vi "WinHostTocRIO.vi"() -> ()   [LabVIEW 2013]
uses:
  <vilib>/userdefined/High Color/nirio_resource_hc.ctl
  <vilib>/nisyscfg/Find Hardware.vi
  <vilib>/nisyscfg/Close (System).vi
  <vilib>/FPGAPlugInAG/NI 9159/niLvFpga_Open_NI 9159.vi
  <vilib>/rvi/interface/common/dynamic/niFpgaDynamicAddResources.vi
  <vilib>/FPGAPlugInAG/Dynamic/niLvFpga_Reset_Dynamic.vi
  <vilib>/FPGAPlugInAG/Dynamic/niLvFpga_Run_Dynamic.vi
  <vilib>/rvi/interface/common/niFpgaWaitOnOcc.vi
  <vilib>/Utility/error.llb/Error Cluster From Error Code.vi
  <vilib>/rvi/errors/niLvFpgaAdjustHostInterfaceError.vi
  <vilib>/FPGAPlugInAG/Dynamic/niLvFpga_Close_Dynamic.vi
  <vilib>/rvi/interface/nirviOpenFPGA/nirviOpenFPGA.xnode
  FPGA Bitfiles/cRIO9159_cRIOIO_v1_1.lvbitx
  cRIO9159_IO.vi
  <vilib>/rvi/interface/nirviMethod/nirviMethod.xnode
  <vilib>/rvi/interface/nirviReadWriteControl/nirviReadWriteControl.xnode
  <vilib>/rvi/interface/nirviCloseFPGA/nirviCloseFPGA.xnode
  <vilib>/rvi/interface/Simulation/niFpgaSimulationCallBeginRW.vi
  NiFpgaLv.dll
  <vilib>/nisyscfg/nisyscfg.lvlib
  <resource>/objmgr/nisysapi.rc
panel:
  out "resource name":T1
  out "Resource":string="RIO0"
  out "resources out":refnum<k20>[](array[refnum])
  in  "stop":bool
  out "error out":errorcluster
  out "Waveform Chart":cluster{ext, ext, ext}(graph)={-0.0011014938354492188, -0.0004444122314453125, -0.0007729530334472656}
  in  "Tab Control":T2(tab)=enum."Optional Resources"
  out "FPGAVIversion":u8[](array[numeric])
  out "InsertedIOModulesID":u16[](array[numeric]) format="%x"
  out "InitDone":bool
  out "cRIOModulesOK":bool
  in  "DebugMode":bool
  out "DevQualityStatus":u8
  out "DeviceTemp":sgl format="%#1.3f"
  out "DevProfile":u8
  out "Fref":u32
  in  "DAQStartStop":bool
  in  "Desired Sampling Rate":dbl=1000.0
  out "SamplingRate":dbl
  in  "AO0":fxp<+/-,20,5>
  in  "AO1":fxp<+/-,20,5>
  in  "AO2":fxp<+/-,20,5>
  in  "AOEnable0":bool
  in  "AOEnable1":bool
  in  "AOEnable2":bool
  out "Numeric":i32=95288553
  in  "auxAO0":i32
  in  "auxAO1":i32
  out "auxAI0":i32
  out "auxAI1":i32
  in  "DO0":bool
  in  "DO1":bool
  in  "DO2":bool
  in  "auxDO0":bool
  in  "auxDO1":bool
  out "DI1":bool
  out "DI2":bool
  out "DI0":bool
  out "auxDI0":bool
  out "auxDI1":bool
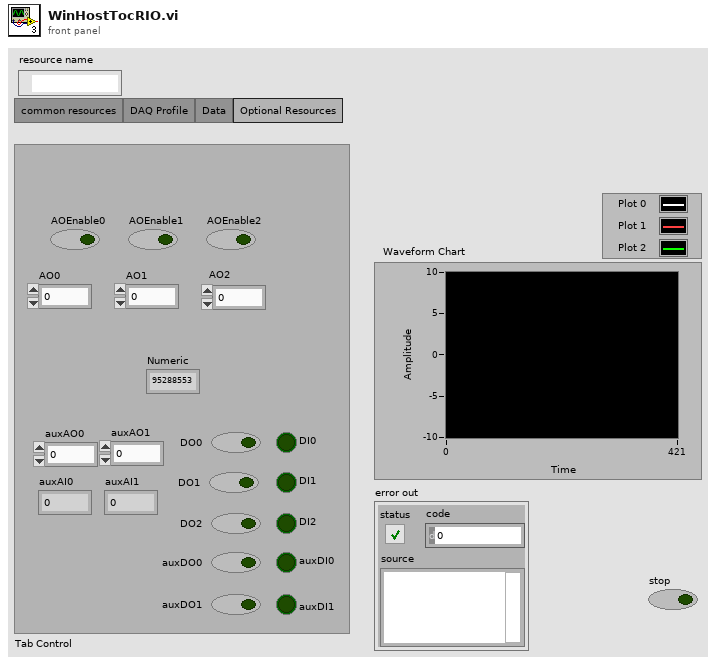
[diagram p1: front panel]
types:
  T1 = typedef "nirio_resource_hc.ctl" = tag
  T2 = enum32{"common resources", "DAQ Profile", "Data", "Optional Resources"}
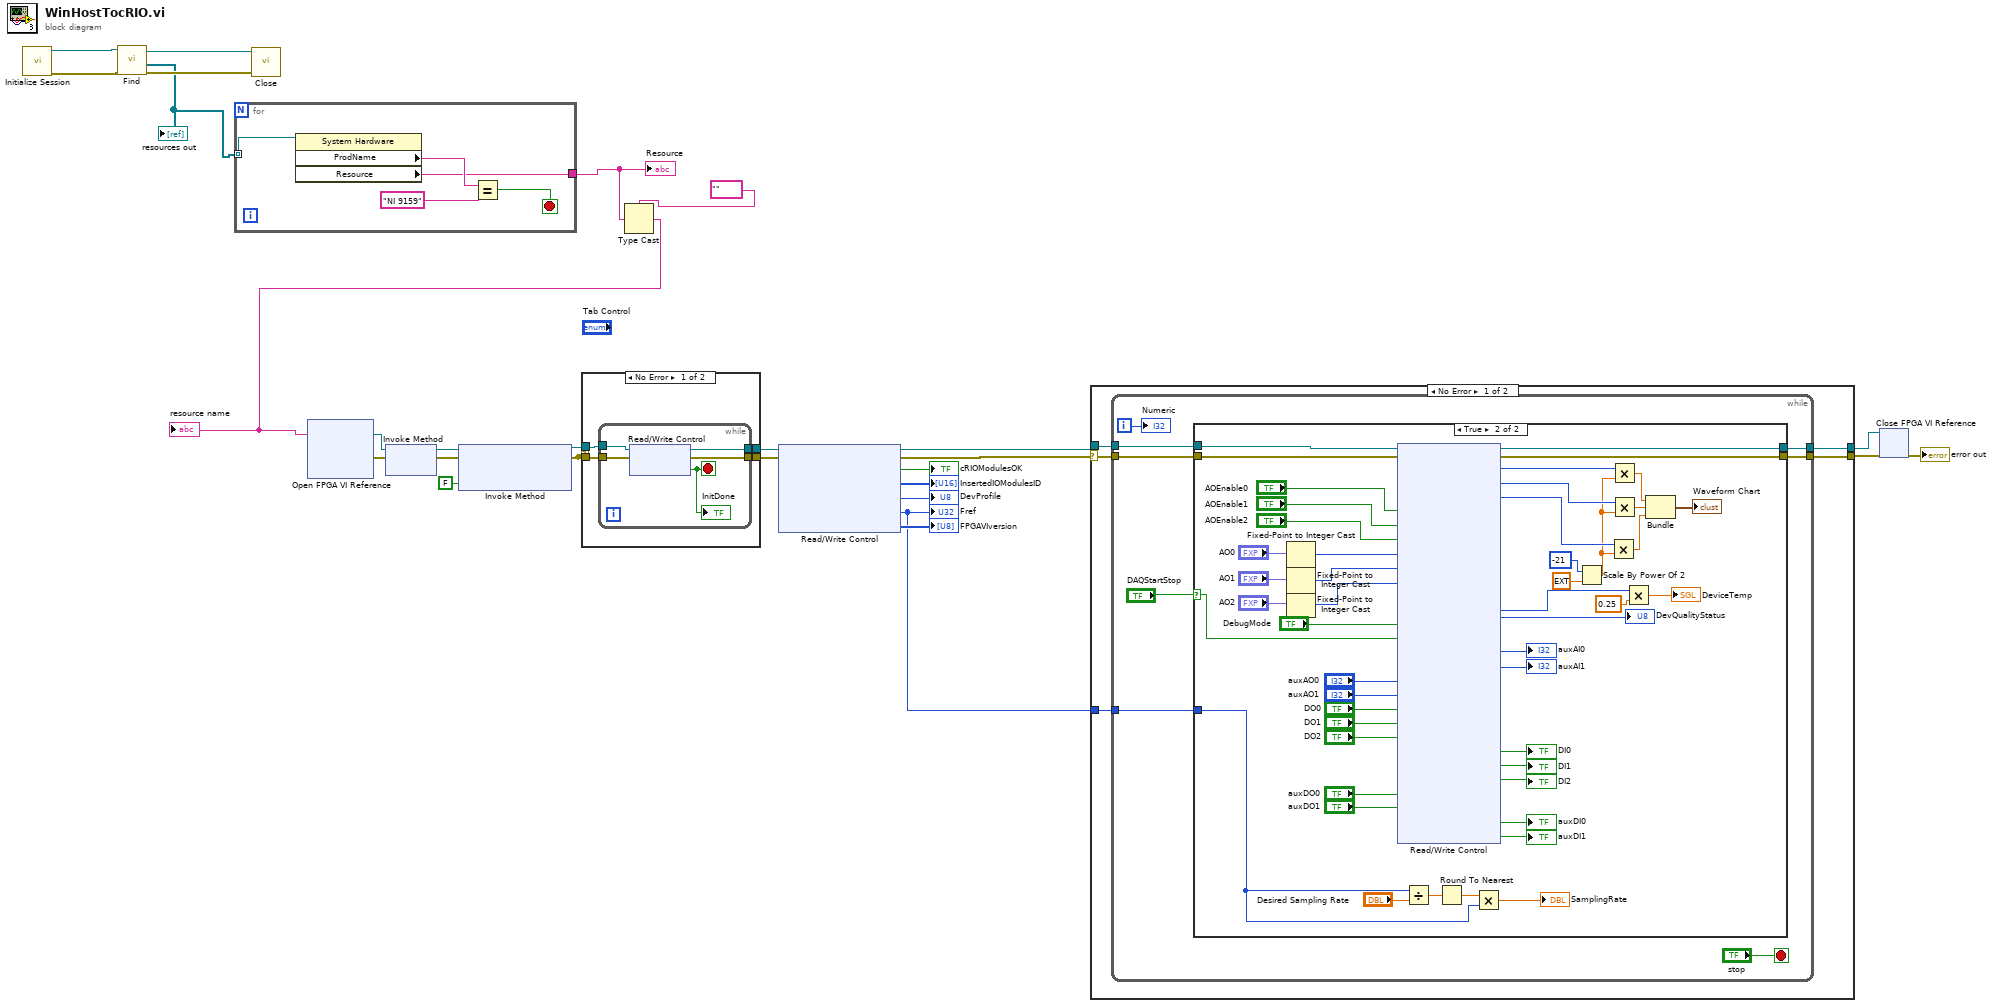
[diagram p0: block diagram]
diagram:
  n1 = call <vilib>:"Initialize Session.vi"() -> ("error out"=w7:errorcluster, "session out"=w8:refnum<k21>)  [unwired: 10 in]
  n2 = call-poly <vilib>:"Find.vi"("error in (no error)"=w7, "session in"=w8) -> ("error out"=w5:errorcluster, "resources out"=w4:refnum<k20>[], "session out"=w6:refnum<k21>)  [unwired: 6 in, 1 out]
  "resources out" <- w4
  n3 = for {
    tunnel: w4 -> [w32] mode=indexing
    tunnel: [w28] -> w3
    stop <- w29 stop-if-true
    n4 = property class="System Hardware"(reference=w32) -> ("ProdName"=w30:string, "Resource"=w28:string)  [unwired: 1 in, 2 out]
    n5 = Equal?(x=w30, y="NI 9159") -> (x = y?=w29:bool)
  }
  "Resource" <- w3
  n6 = call-poly <vilib>:"Close.vi"("error in (no error)"=w5, "session in"=w6) -> ()  [unwired: 9 in, 1 out]
  n7 = Type Cast(type=T1 "" ("resource name 2"), x=w3) -> (*(type *) &x=w1:T1)
  "resource name" <- w1
  n8 = xnode "Open FPGA VI Reference"("resource name"=w1) -> ("FPGA VI Reference Out"=w23:refnum<k20>, "error out"=w24:errorcluster)  [unwired: 1 in]
  n9 = xnode "Invoke Method"("FPGA VI Reference In"=w23, "error in"=w24) -> ("FPGA VI Reference Out"=w27:refnum<k20>, "error out"=w26:errorcluster)
  n10 = xnode "Invoke Method"("FPGA VI Reference In"=w27, "error in"=w26, "Wait Until Done (F)"=FALSE) -> ("FPGA VI Reference Out"=w22:refnum<k20>, "error out"=w18:errorcluster)
  n11 = case shown="No Error" w18 {
    tunnel: [w36 w42] -> w17
    tunnel: w22 -> [w35 w42]
    tunnel: [w34 w43] -> w16
    tunnel: w18 -> [w33 w43]
    frame No Error {
      n12 = while {
        tunnel: w35 -> [w41]
        tunnel: w33 -> [w40]
        tunnel: [w38] -> w36
        tunnel: [w37] -> w34
        stop <- w39 stop-if-true
        n13 = xnode "Read/Write Control"("FPGA VI Reference In"=w41, "error in"=w40) -> ("FPGA VI Reference Out"=w38:refnum<k20>, "error out"=w37:errorcluster, "InitDone"=w39:bool)
        "InitDone" <- w39
      }
    }
    frame Error {
    }
  }
  n14 = xnode "Read/Write Control"("FPGA VI Reference In"=w17, "error in"=w16) -> ("FPGA VI Reference Out"=w11:refnum<k20>, "error out"=w12:errorcluster, "cRIOModulesOK"=→"cRIOModulesOK":bool, "InsertedIOModulesID"=→"InsertedIOModulesID":u16[], "DevProfile"=→"DevProfile":u8, "Fref"=w9:u32, "FPGAVIversion"=→"FPGAVIversion":u8[])
  "Fref" <- w9
  n15 = case shown="No Error" w12 {
    selector: w12 -> [w45 w107]
    tunnel: [w48 w108] -> w21
    tunnel: [w47 w107] -> w20
    tunnel: w11 -> [w46 w108]
    tunnel: w9 -> [w44 _]
    frame No Error {
      n16 = while {
        tunnel: [w54] -> w48
        tunnel: [w53] -> w47
        tunnel: w46 -> [w52]
        tunnel: w45 -> [w51]
        tunnel: w44 -> [w49]
        i -> [w55]
        stop <- "stop" stop-if-true
        n17 = case shown="True" "DAQStartStop" {
          selector: "DAQStartStop" -> [_ w76]
          tunnel: [w57 w91] -> w54
          tunnel: [w58 w90] -> w53
          tunnel: w52 -> [w57 w81]
          tunnel: w51 -> [w58 w80]
          tunnel: w49 -> [_ w78]
          frame False {
          }
          frame True {
            n18 = Fixed-Point to Integer Cast(1:"AO0") -> (0:w94:i32)
            n19 = Fixed-Point to Integer Cast(1:"AO1") -> (0:w93:i32)
            n20 = Fixed-Point to Integer Cast(1:"AO2") -> (0:w92:i32)
            n21 = xnode "Read/Write Control"("FPGA VI Reference In"=w81, "error in"=w80, "AOEnable0"="AOEnable0", "AOEnable1"="AOEnable1", "AOEnable2"="AOEnable2", "AO0"=w94, "AO1"=w93, "AO2"=w92, "DebugMode"="DebugMode", "DAQStartStop"=w76, "auxAO0"="auxAO0", "auxAO1"="auxAO1", "DO0"="DO0", "DO1"="DO1", "DO2"="DO2", "auxDO0"="auxDO0", "auxDO1"="auxDO1") -> ("FPGA VI Reference Out"=w91:refnum<k20>, "error out"=w90:errorcluster, "AI0"=w89:i32, "AI1"=w88:i32, "AI2"=w87:i32, "DevQualityStatus"=→"DevQualityStatus":u8, "DevTemp"=w74:i16, "auxAI0"=→"auxAI0":i32, "auxAI1"=→"auxAI1":i32, "DI0"=→"DI0":bool, "DI1"=→"DI1":bool, "DI2"=→"DI2":bool, "auxDI0"=→"auxDI0":bool, "auxDI1"=→"auxDI1":bool)
            n22 = Divide(x=w78, y="Desired Sampling Rate") -> (x/y=w105:dbl)
            n23 = Round To Nearest(number=w105) -> (nearest integer value=w104:dbl)
            n24 = Multiply(x=w104, y=w78) -> (x*y=→"SamplingRate":dbl)
            n25 = Scale By Power Of 2(n=i16 -21, x=ext 1.0) -> (x*2^n=w86:ext)
            n26 = Multiply(x=w87, y=w86) -> (x*y=w83:ext)
            n27 = Multiply(x=w89, y=w86) -> (x*y=w85:ext)
            n28 = Multiply(x=w88, y=w86) -> (x*y=w84:ext)
            n29 = Multiply(x=w74, y=sgl 0.25) -> (x*y=→"DeviceTemp":sgl)
            n30 = Bundle(w85, w84, w83) -> (→"Waveform Chart":cluster{ext, ext, ext})  [unwired: 1 in]
          }
        }
        "Numeric" <- w55
      }
    }
    frame Error {
    }
  }
  n31 = xnode "Close FPGA VI Reference"("FPGA VI Reference In"=w21, "error in"=w20) -> ("error out"=→"error out":errorcluster)
